vi "SetSpeed.vi"(0 "VRN IN":refnum<visa-resource-name>, 5 "Axis Number":u8=1 min=1 max=4 step=1, 7 "Low Speed":u32=100 min=1 max=500000, 9 "High Speed":u32=1000 min=1 max=500000, 11 "Acceleration Time":u32=100 max=1000) -> (4 "VRN OUT":refnum<visa-resource-name>, 8 "OK Done":bool, 15 "error out":errorcluster)   [LabVIEW 2019]
panel:
  # "Port Number 0=COM1"
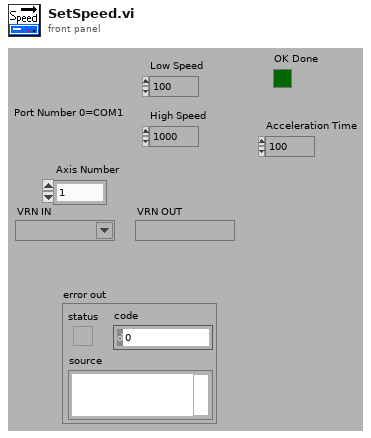
[diagram p1: front panel]
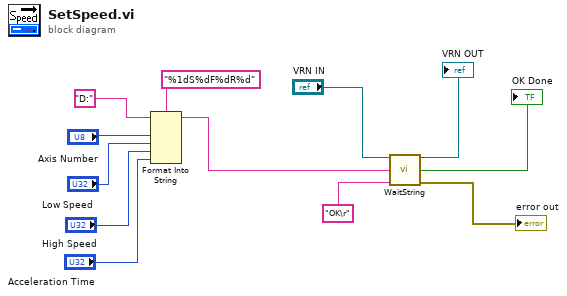
[diagram p0: block diagram]
diagram:
  n1 = Format Into String(format string="%1dS%dF%dR%d", initial string="D:", "Axis Number", "Low Speed", "High Speed", "Acceleration Time") -> (resulting string=w6:string)  [unwired: 1 in, 1 out]
  n2 = call "WaitString.vi"("reference"="VRN IN", "String to Send"=w6, "String to Receive"="OK\r") -> ("reference dup"=→"VRN OUT":refnum<visa-resource-name>, "OK Done"=→"OK Done":bool, "error out"=→"error out":errorcluster)  [unwired: 10 in]
